vi "pulse pixel.vi"   [LabVIEW 2018, in "state machine.lvlib"]
uses:
  state machine.lvlib
  <vilib>/rvi/eio/common/nirviEmuTemplateMethod_errors.vi
  <vilib>/eio/EIONode/EIONode.xnode
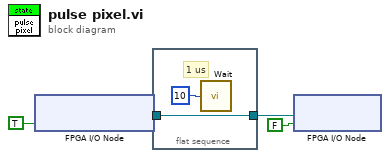
[diagram p0: block diagram]
diagram:
  n1 = xnode "FPGA I/O Node"("pixel clock out"=TRUE ("smaract out")) -> ("FPGA I/O Out"=w3:refnum<k21>)  [unwired: 1 in]
  n2 = flat-sequence {
    tunnel: w3 -> [w6]
    tunnel: [w6] -> w4
    frame #0 {
      # "1 us"
      n3 = call "Wait"("Count(uSec)"=u32 10) -> ()  [unwired: 1 out]
    }
  }
  n4 = xnode "FPGA I/O Node"("I/O Item"=FALSE ("smaract out"), "FPGA I/O In"=w4) -> ()  [unwired: 1 out]
